vi "Check Ack_Nack.vi"(8 "error in (no error)":errorcluster, 11 "Low Speed in":refnum<class "Low Speed.lvclass">) -> (0 "error out":errorcluster, 3 "Low Speed out":refnum<class "Low Speed.lvclass">)   [LabVIEW 2020]
uses:
  Low Speed.lvclass
  C:/Users/kaiser.asan/OneDrive - SolitonTechnologies/LabVIEW/29.SDLC - I2C Driver/I2C Module/I2C Controller Module/Class/Transmission Mode/Parent/TX Speed.lvclass
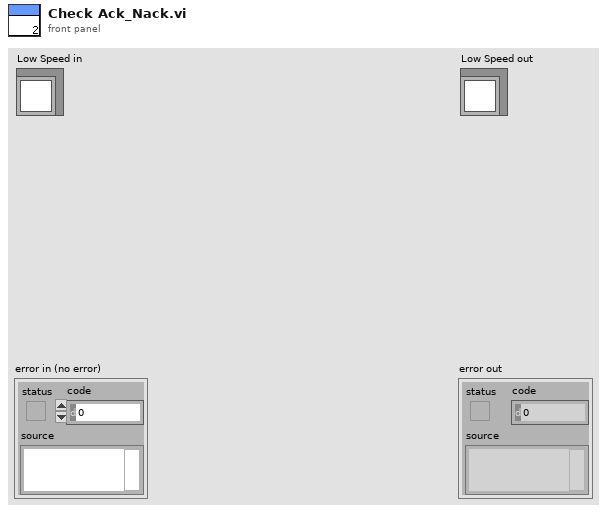
[diagram p1: front panel]
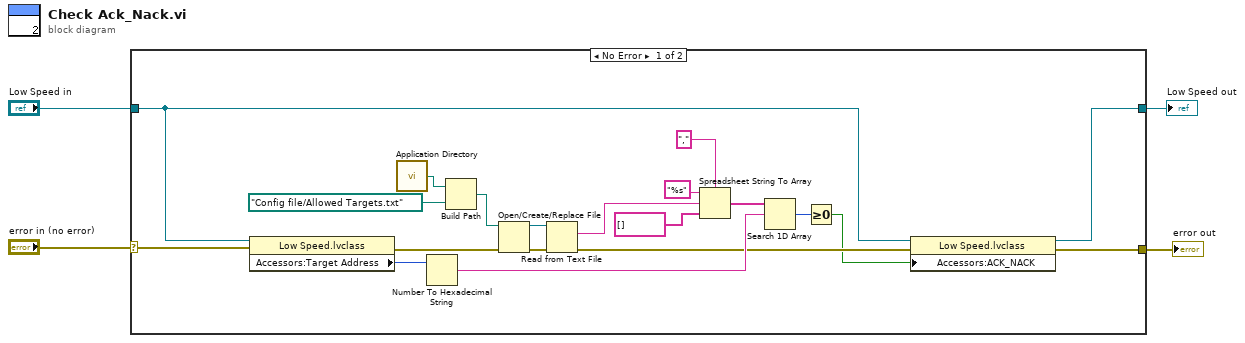
[diagram p0: block diagram]
diagram:
  n1 = case shown="No Error" "error in (no error)" {
    selector: "error in (no error)" -> [w10 w26]
    tunnel: [w8 w26] -> w3
    tunnel: [w6 w25] -> w1
    tunnel: "Low Speed in" -> [w7 w25]
    frame No Error {
      n2 = property class="Low Speed.lvclass"(reference=w7, error in=w10) -> (error out=w22:errorcluster, "Accessors:Target Address"=w15:u16)  [unwired: 1 out]
      n3 = call <vilib>:"Application Directory.vi"() -> ("Application Directory"=w24:path)
      n4 = Number To Hexadecimal String(2:w15) -> (0:w14:string)  [unwired: 1 in]
      n5 = Build Path(base path=w24, name or relative path=path "Config file/Allowed Targets.txt" ("Application Directory")) -> (appended path=w21:path)
      n6 = Open/Create/Replace File(file path (use dialog)=w21, error in=w22) -> (refnum out=w19:refnum<file>, error out=w20:errorcluster)  [unwired: 4 in, 1 out]
      n7 = Read from Text File(file (use dialog)=w19, error in=w20) -> (text=w18:string, error out=w9:errorcluster)  [unwired: 2 in, 2 out]
      n8 = Spreadsheet String To Array(delimiter (Tab)=",", format string="%s", spreadsheet string=w18, array type (2D Dbl)=string[] [] ("text")) -> (array=w16:string[])
      n9 = Search 1D Array(1D array=w16, element=w14) -> (index of element=w13:i32)  [unwired: 1 in]
      n10 = Greater Or Equal To 0?(x=w13) -> (x >= 0?=w5:bool)
      n11 = property class="Low Speed.lvclass"(reference=w7, error in=w9, "Accessors:ACK_NACK"=w5) -> (reference out=w6:refnum<class "Low Speed.lvclass">, error out=w8:errorcluster)
    }
    frame Error {
    }
  }
  "error out" <- w3
  "Low Speed out" <- w1
